vi "rwfm_AcqConfig(Ss).vi"(5 "Samples per Channel":i32=1000, 7 "Sample Mode":enum16{"Finite Samples", "Continuous Samples"}(ring), 8 "error in":errorcluster, 9 "Sample Rate S/s":u32, 10 "Sampling Info In":T2, 11 "Dynamic FPGA Ref":T1) -> (0 "error out":errorcluster, 1 "Buffer Size [Total Samples]":u32, 2 "Sampling Info Out":T2, 3 "Dynamic FPGA Ref Out":T1)   [LabVIEW 2017, in "cRIOWfmLibMcsa.lvlib"]
doc: "This VI sets the sampling mode (either finite or continuous) and transfers sampling rate to the FPGA. Pay close attention to the polymorphic instance used by this VI. Some NI C Series modules support sample rates that are integer divisions of 51.2 kS/s and some support sample rates that are integer divisions of 50 kS/s. When you synchronize multiple Delta Sigma modules together, the supported rates of all modules are equal to the supported rates of the master. Timebase sharing is configured through the LabVIEW project.\n\nIf the overall data rate is not dictated by a Delta Sigma-based C Series module, be sure to select the \"Non Delta Sigma\" instance of this VI."
uses:
  <vilib>/addons/InsightCM/Devices/Shared/Mcsa/cRIOWfmAcqMcsa/cRIOWfmLibMcsa.lvlib
  <vilib>/addons/InsightCM/Devices/Shared/Cms/cRIOWfmAcq/subVIs/RIO Wfm Cust Ctrls/rwfm_SamplingInfo.ctl
  <vilib>/addons/InsightCM/Devices/Shared/Mcsa/cRIOWfmAcqMcsa/controls/rwfm_DynamicFPGArefMCSA.ctl
  <vilib>/Utility/error.llb/Error Cluster From Error Code.vi
  <vilib>/rvi/errors/niLvFpgaAdjustHostInterfaceError.vi
  <vilib>/rvi/interface/nirviReadWriteControl/nirviReadWriteControl.xnode
  NiFpgaLv.dll
  <vilib>/rvi/interface/Simulation/niFpgaSimulationCallBeginRW.vi
  <vilib>/addons/InsightCM/Devices/Shared/Cms/cRIOWfmAcq/cRIOWfmLib.lvlib
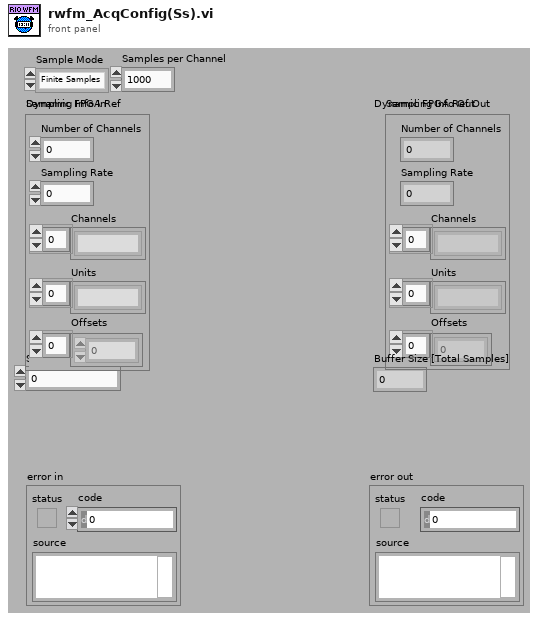
[diagram p1: front panel]
types:
  T1 = typedef "cRIOWfmLibMcsa.lvlib/rwfm_DynamicFPGArefMCSA.ctl" = refnum<k20>
  T2 = typedef "cRIOWfmLib.lvlib/rwfm_SamplingInfo.ctl" = cluster{"Number of Channels":i32, "Sampling Rate":dbl, "Channels":string[], "Units":string[], "Offsets":sgl[]}
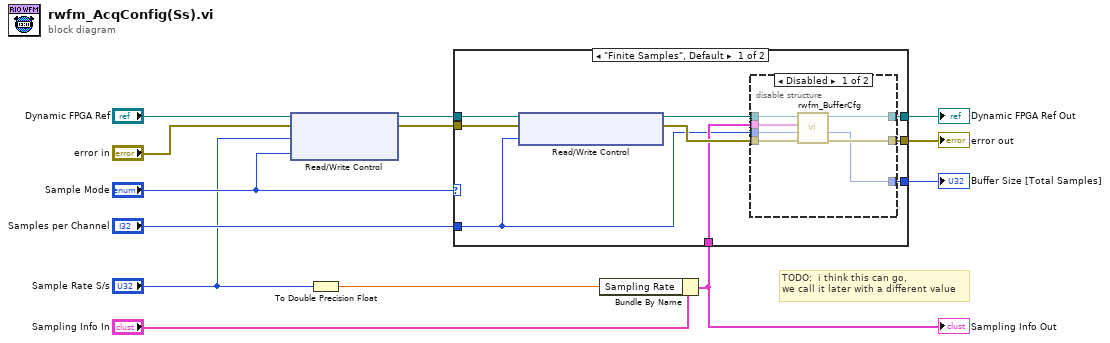
[diagram p0: block diagram]
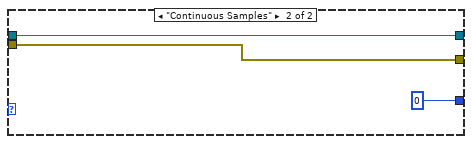
[diagram p3: hidden frame]
diagram:
  # "TODO:  i think this can go, \nwe call it later with a different value"
  n1 = xnode "Read/Write Control"("FPGA VI Reference In"="Dynamic FPGA Ref", "error in"="error in", "Data Rate [S/s]"="Sample Rate S/s", "Acquisition Type"="Sample Mode") -> ("FPGA VI Reference Out"=w13:T1, "error out"=w12:errorcluster)
  n2 = To Double Precision Float(number="Sample Rate S/s") -> (double precision float=w3:dbl)
  n3 = Bundle By Name(cluster="Sampling Info In", "Sampling Rate"=w3) -> (w8:T2)
  "Sampling Info Out" <- w8
  n4 = case shown="\"Finite Samples\", Default" "Sample Mode" {
    tunnel: w13 -> [w22 w32]
    tunnel: w12 -> [w21 w31]
    tunnel: [w14 w32] -> w4
    tunnel: [w19 w31] -> w9
    tunnel: w8 -> [w18 _]
    tunnel: "Samples per Channel" -> [w17 _]
    tunnel: [w16 u32 0 ("Buffer Size [Total Samples]")] -> w6
    frame "Finite Samples", Default {
      n5 = xnode "Read/Write Control"("FPGA VI Reference In"=w22, "error in"=w21, "Samps per Chan [Finite]"=w17) -> ("FPGA VI Reference Out"=w15:T1, "error out"=w20:errorcluster)
      n6 = disable-structure shown="Disabled" {
        disable-tunnel: w20 -> [w29 _]
        disable-tunnel: [w28 _] -> w19
        disable-tunnel: w18 -> [w27 _]
        disable-tunnel: w17 -> [w26 _]
        disable-tunnel: [w25 _] -> w16
        disable-tunnel: w15 -> [w24 w30]
        disable-tunnel: [w23 w30] -> w14
        frame Disabled {
          n7 = call <vilib>:"rwfm_BufferCfg.vi"("error in"=w29, "Buffer Size [Samps per Chan]"=w26, "Sampling Info In"=w27, "Dynamic FPGA VI Reference"=w24) -> ("error out"=w28:errorcluster, "Buffer Size [Total Samples]"=w25:u32, "Dynamic FPGA VI Reference"=w23:T1)  [unwired: 4 in, 1 out]
        }
        frame Enabled {
        }
      }
    }
    frame "Continuous Samples" {
    }
  }
  "error out" <- w9
  "Buffer Size [Total Samples]" <- w6
  "Dynamic FPGA Ref Out" <- w4
